vi "PAN_ActionsMgr.vi"(10 "id":string) -> ()   [LabVIEW 2016]
panel:
  out "Array":T1(array[cluster])
  in  "Cluster":T2
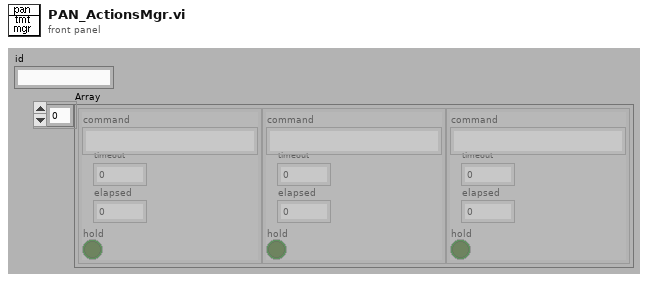
[diagram p1: front panel]
types:
  T1 = cluster{"command":string, "timeout":i32, "elapsed":i32, "hold":bool}[]
  T2 = cluster{"command":string, "timeout":i32, "elapsed":i32, "hold":bool}
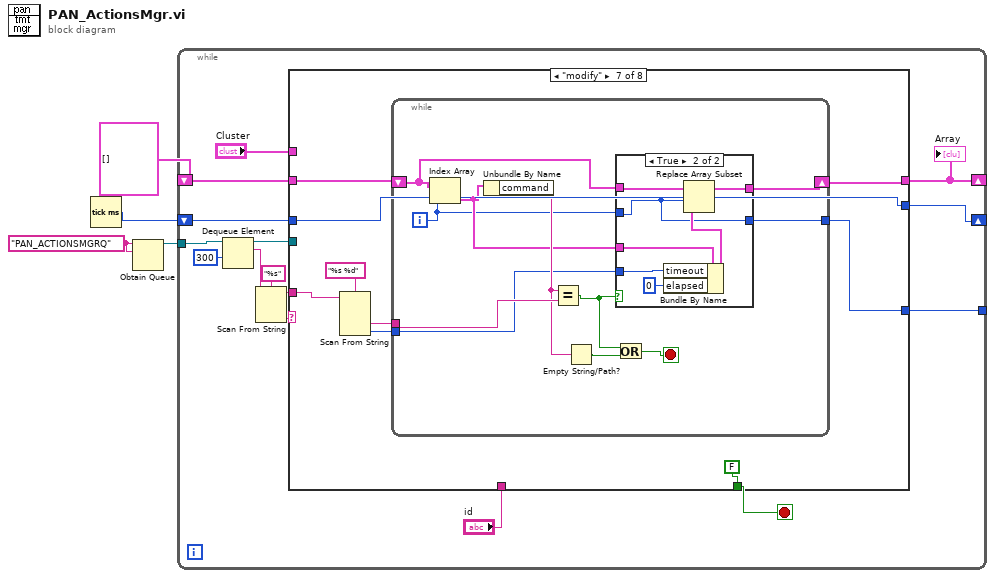
[diagram p0: block diagram]
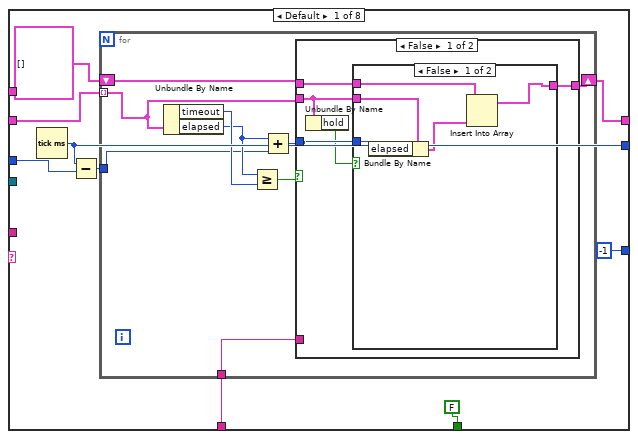
[diagram p2: hidden frame]
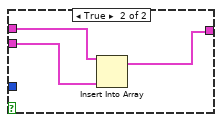
[diagram p3: hidden frame]
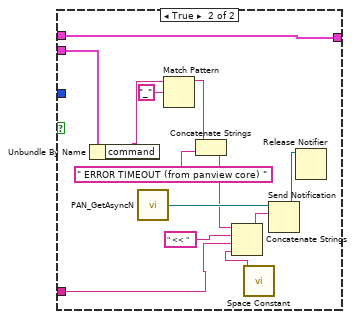
[diagram p4: hidden frame]
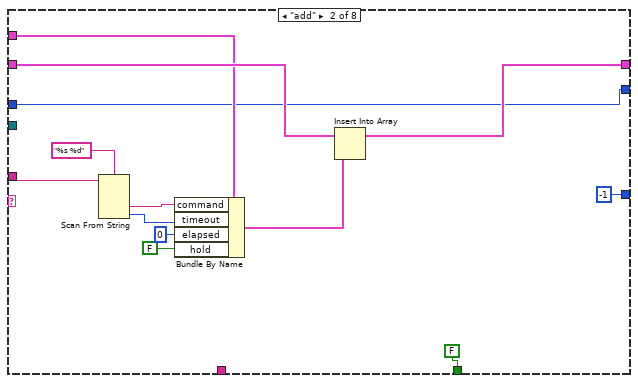
[diagram p5: hidden frame]
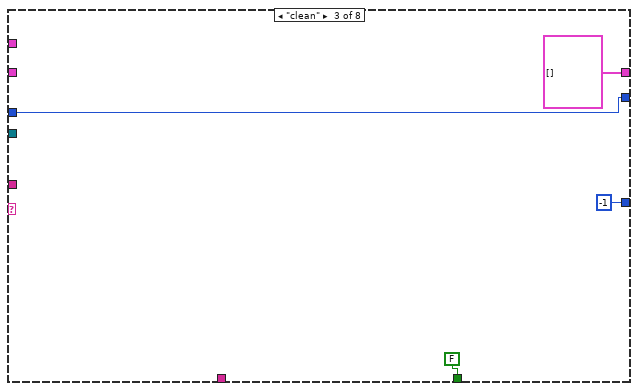
[diagram p6: hidden frame]
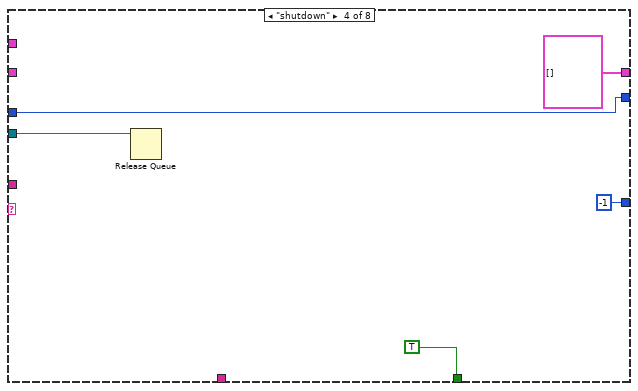
[diagram p7: hidden frame]
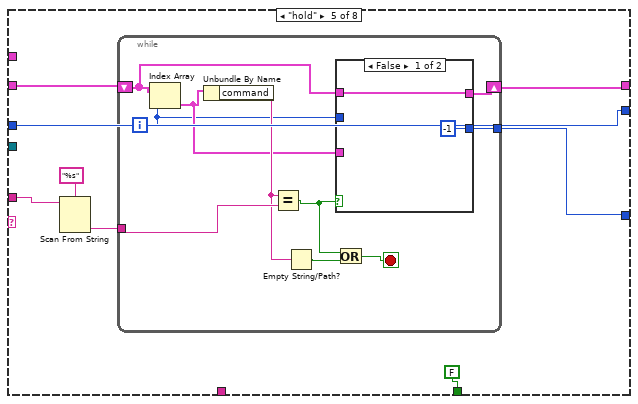
[diagram p8: hidden frame]
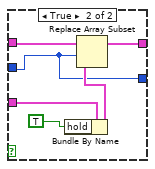
[diagram p9: hidden frame]
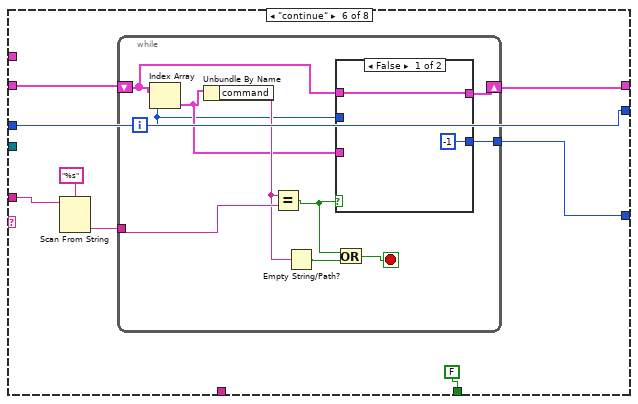
[diagram p10: hidden frame]
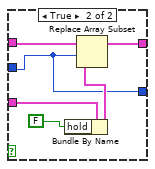
[diagram p11: hidden frame]
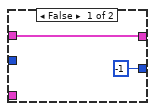
[diagram p12: hidden frame]
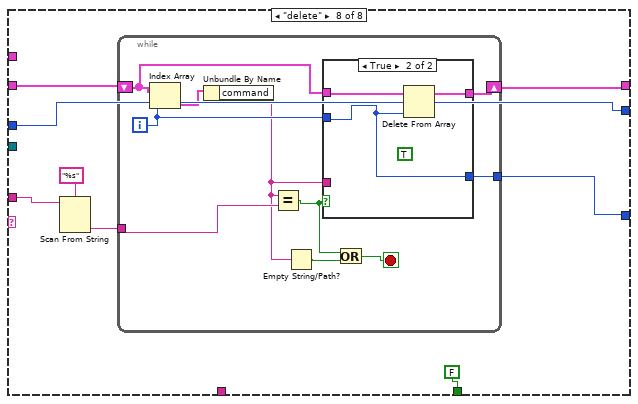
[diagram p13: hidden frame]
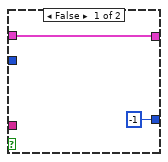
[diagram p14: hidden frame]
diagram:
  w3 = "PAN_ACTIONSMGRQ" ("name (unnamed)")
  n1 = Tick Count (ms)() -> (millisecond timer value=w2:u32)
  n2 = Obtain Queue(name (unnamed)=w3, element data type=w3) -> (queue out=w4:refnum<queue>)  [unwired: 3 in, 2 out]
  n3 = while {
    tunnel: w4 -> [w19]
    shift-right: [w12] -> _
    shift-left: T1 [] -> [w11]
    shift-right: [w6] -> _
    shift-left: w2 -> [w8]
    tunnel: [w7] -> _
    stop <- w15 stop-if-true
    n4 = Dequeue Element(queue=w19, timeout in ms (-1)=300) -> (queue out=w9:refnum<queue>, element=w18:string)  [unwired: 1 in, 2 out]
    n5 = Scan From String(format string="%s", input string=w18) -> (remaining string=w13:string, output 1=w16:string)  [unwired: 2 in, 3 out]
    n6 = case shown="\"modify\"" w16 {
      tunnel: [FALSE FALSE FALSE TRUE FALSE FALSE FALSE FALSE] -> w15
      tunnel: w13 -> [_ w75 _ _ w93 w119 w146 w174]
      tunnel: [w26 w73 T1 [] T1 [] w88 w114 w141 w169] -> w12
      tunnel: w11 -> [w27 w72 _ _ w89 w115 w142 w170]
      tunnel: "Cluster" -> [_ w71 _ _ _ _ _ _]
      tunnel: w9 -> [_ _ _ w84 _ _ _ _]
      tunnel: w8 -> [w25 w66 w77 w81 w86 w112 w138 w167]
      tunnel: [-1 -1 -1 -1 w87 w113 w139 w168] -> w7
      tunnel: [w21 w66 w77 w81 w86 w112 w138 w167] -> w6
      tunnel: "id" -> [w20 _ _ _ _ _ _ _]
      frame Default {
        n7 = Tick Count (ms)() -> (millisecond timer value=w21:u32)
        n8 = Subtract(x=w21, y=w25) -> (x-y=w24:u32)
        n9 = for {
          tunnel: w27 -> [w37] mode=indexing
          shift-right: [w36] -> w26
          shift-left: T1 [] -> [w35]
          tunnel: w24 -> [w31]
          tunnel: w20 -> [w29]
          n10 = Unbundle By Name(w37) -> ("timeout"=w34:i32, "elapsed"=w32:i32)
          n11 = Greater Or Equal?(x=w32, y=w34) -> (x >= y?=w33:bool)
          n12 = Add(x=w32, y=w31) -> (x+y=w30:u32)
          n13 = case shown="False" w33 {
            tunnel: w37 -> [w39 w63]
            tunnel: w35 -> [w42 w62]
            tunnel: [w41 w62] -> w36
            tunnel: w30 -> [w40 _]
            tunnel: w29 -> [_ w54]
            frame False {
              n14 = Unbundle By Name(w39) -> ("hold"=w38:bool)
              n15 = case shown="False" w38 {
                tunnel: w39 -> [w47 w50]
                tunnel: w42 -> [w46 w48]
                tunnel: [w44 w49] -> w41
                tunnel: w40 -> [w43 _]
                frame False {
                  n16 = Bundle By Name(cluster=w47, "elapsed"=w43) -> (w45:T2)
                  n17 = Insert Into Array(array=w46, new element=w45) -> (w44:T1)  [unwired: 1 in]
                }
                frame True {
                  n18 = Insert Into Array(array=w48, new element=w50) -> (w49:T1)  [unwired: 1 in]
                }
              }
            }
            frame True {
              n19 = Unbundle By Name(w63) -> ("command"=w53:string)
              n20 = call "PAN_GetAsyncN.vi"() -> ("asyncN"=w61:refnum<notifier>)  [unwired: 11 out]
              n21 = Match Pattern(string=w53, regular expression="_") -> (before substring=w51:string)  [unwired: 4 out]
              n22 = Concatenate Strings(w51, " ERROR TIMEOUT (from panview core) ") -> (w55:string)
              n23 = call <vilib>:"Space Constant.vi"() -> ("String"=w57:string)
              n24 = Concatenate Strings(w55, " << " ("string"), w54, w57) -> (w56:string)
              n25 = Send Notification(notification=w56, notifier=w61) -> (notifier out=w60:refnum<notifier>)  [unwired: 1 in, 1 out]
              n26 = Release Notifier(notifier=w60) -> ()  [unwired: 1 in, 4 out]
            }
          }
        }
      }
      frame "add" {
        n27 = Scan From String(format string="%s %d", input string=w75) -> (output 1=w65:string, output 2=w64:i32)  [unwired: 2 in, 5 out]
        n28 = Bundle By Name(cluster=w71, "command"=w65, "timeout"=w64, "elapsed"=0, "hold"=FALSE) -> (w70:T2)
        n29 = Insert Into Array(array=w72, new element=w70) -> (w73:T1)  [unwired: 1 in]
      }
      frame "clean" {
      }
      frame "shutdown" {
        n30 = Release Queue(queue=w84) -> ()  [unwired: 1 in, 4 out]
      }
      frame "hold" {
        n31 = Scan From String(format string="%s", input string=w93) -> (output 1=w90:string)  [unwired: 2 in, 4 out]
        n32 = while {
          tunnel: w90 -> [w103]
          shift-right: [w95] -> w88
          shift-left: w89 -> [w97]
          tunnel: [w94] -> w87
          i -> [w96]
          stop <- w102 stop-if-true
          n33 = Index Array(array=w97, index=w96) -> (element=w98:T2)
          n34 = Unbundle By Name(w98) -> ("command"=w101:string)
          n35 = Equal?(x=w101, y=w103) -> (x = y?=w99:bool)
          n36 = Empty String/Path?(string/path=w101) -> (empty?=w100:bool)
          n37 = case shown="False" w99 {
            tunnel: w98 -> [_ w110]
            tunnel: w97 -> [w105 w109]
            tunnel: w96 -> [_ w106]
            tunnel: [w105 w107] -> w95
            tunnel: [-1 w106] -> w94
            frame False {
            }
            frame True {
              n38 = Bundle By Name(cluster=w110, "hold"=TRUE) -> (w108:T2)
              n39 = Replace Array Subset(array=w109, new element=w108, index=w106) -> (w107:T1)
            }
          }
          n40 = Or(x=w99, y=w100) -> (x .or. y?=w102:bool)
        }
      }
      frame "continue" {
        n41 = Scan From String(format string="%s", input string=w119) -> (output 1=w116:string)  [unwired: 2 in, 4 out]
        n42 = while {
          tunnel: w116 -> [w129]
          shift-right: [w121] -> w114
          shift-left: w115 -> [w123]
          tunnel: [w120] -> w113
          i -> [w122]
          stop <- w128 stop-if-true
          n43 = Index Array(array=w123, index=w122) -> (element=w124:T2)
          n44 = Unbundle By Name(w124) -> ("command"=w127:string)
          n45 = Equal?(x=w127, y=w129) -> (x = y?=w125:bool)
          n46 = Empty String/Path?(string/path=w127) -> (empty?=w126:bool)
          n47 = case shown="False" w125 {
            tunnel: w124 -> [_ w136]
            tunnel: w123 -> [w131 w135]
            tunnel: w122 -> [_ w132]
            tunnel: [w131 w133] -> w121
            tunnel: [-1 w132] -> w120
            frame False {
            }
            frame True {
              n48 = Bundle By Name(cluster=w136, "hold"=FALSE) -> (w134:T2)
              n49 = Replace Array Subset(array=w135, new element=w134, index=w132) -> (w133:T1)
            }
          }
          n50 = Or(x=w125, y=w126) -> (x .or. y?=w128:bool)
        }
      }
      frame "modify" {
        n51 = Scan From String(format string="%s %d", input string=w146) -> (output 1=w143:string, output 2=w140:i32)  [unwired: 2 in, 5 out]
        n52 = while {
          tunnel: w143 -> [w157]
          shift-right: [w149] -> w141
          shift-left: w142 -> [w151]
          tunnel: w140 -> [w148]
          tunnel: [w147] -> w139
          i -> [w150]
          stop <- w156 stop-if-true
          n53 = Index Array(array=w151, index=w150) -> (element=w152:T2)
          n54 = Unbundle By Name(w152) -> ("command"=w155:string)
          n55 = Equal?(x=w155, y=w157) -> (x = y?=w153:bool)
          n56 = Empty String/Path?(string/path=w155) -> (empty?=w154:bool)
          n57 = case shown="True" w153 {
            tunnel: w152 -> [_ w166]
            tunnel: w151 -> [w159 w165]
            tunnel: w150 -> [_ w161]
            tunnel: [w159 w163] -> w149
            tunnel: w148 -> [_ w162]
            tunnel: [-1 w161] -> w147
            frame False {
            }
            frame True {
              n58 = Bundle By Name(cluster=w166, "timeout"=w162, "elapsed"=0) -> (w164:T2)
              n59 = Replace Array Subset(array=w165, new element=w164, index=w161) -> (w163:T1)
            }
          }
          n60 = Or(x=w153, y=w154) -> (x .or. y?=w156:bool)
        }
      }
      frame "delete" {
        n61 = Scan From String(format string="%s", input string=w174) -> (output 1=w171:string)  [unwired: 2 in, 4 out]
        n62 = while {
          tunnel: w171 -> [w184]
          shift-right: [w177] -> w169
          shift-left: w170 -> [w179]
          tunnel: [w176] -> w168
          i -> [w178]
          stop <- w183 stop-if-true
          n63 = Index Array(array=w179, index=w178) -> (element=w180:T2)
          n64 = Unbundle By Name(w180) -> ("command"=w175:string)
          n65 = Equal?(x=w175, y=w184) -> (x = y?=w181:bool)
          n66 = Empty String/Path?(string/path=w175) -> (empty?=w182:bool)
          n67 = case shown="True" w181 {
            tunnel: w179 -> [w186 w189]
            tunnel: w178 -> [_ w187]
            tunnel: [w186 w188] -> w177
            tunnel: [-1 w187] -> w176
            tunnel: w175 -> [_ _]
            frame False {
            }
            frame True {
              (unwired) TRUE ("append to file? (new file:F)")
              n68 = Delete From Array(array=w189, index=w187) -> (array with subset deleted=w188:T1)  [unwired: 1 in, 1 out]
            }
          }
          n69 = Or(x=w181, y=w182) -> (x .or. y?=w183:bool)
        }
      }
    }
    "Array" <- w12
  }
